vi "Initialize Message.vi"(6 "Parameters":T8[](array[typedef]) {"Base Word" format="%04d"}, 8 "error in (no error)":errorcluster, 10 "Message  Config":T1={"Time to Next Msg (4 us)"=100, "Command Config"={"Command Type"=enum."Transmit", "Terminal Address"=enum."0", "SubAddress"=enum."1", "Word Count\\Mode Code"=enum."1", "Command Data"=[]}, "Message Control"={"MC17 Time Sync"=FALSE, "Error Mask"=FALSE, "Service Request Mask"=FALSE, "Busy Mask"=FALSE, "SubSystem Flag Mask"=FALSE, "Terminal Flag Mask"=FALSE, "Reserved Mask"=FALSE, "Retry"=FALSE, "Bus A / !Bus B"=FALSE, "Self-Test Loopback"=FALSE, "Broadcast Mask"=FALSE, "EoM Interrupt"=FALSE, "Mode Code Format"=FALSE, "Broadcast Format"=FALSE, "RT-RT Format"=FALSE}}, 11 "ID":string) -> (0 "error out":errorcluster, 3 "Message out":refnum<class "Message.lvclass">)   [LabVIEW 2020, in "BCI-1553 API.lvlib" / "Message.lvclass"]
doc: "Generates a Message object that can be added to a Major Frame. Once added to a Major Frame, the Major Frame and all the Minor Frames active in it can all use this Message in their sequences.\n\nEach Message & RT-RT Message requires a unique ID within a single Major Frame."
uses:
  Message.lvclass
  TypeDefs/Simplified Parameter Data Table.ctl
  TypeDefs/Scaling Information.ctl
  TypeDefs/Message Config.ctl
  TypeDefs/Command Config.ctl
  TypeDefs/Command Type.ctl
  TypeDefs/Command Terminal Address.ctl
  TypeDefs/Command SubAddress.ctl
  TypeDefs/Command Word Count.ctl
  TypeDefs/Message Control.ctl
  TypeDefs/Parameter Table Data.ctl
  Message.lvclass/Message.ctl
  BCI-1553 API.lvlib
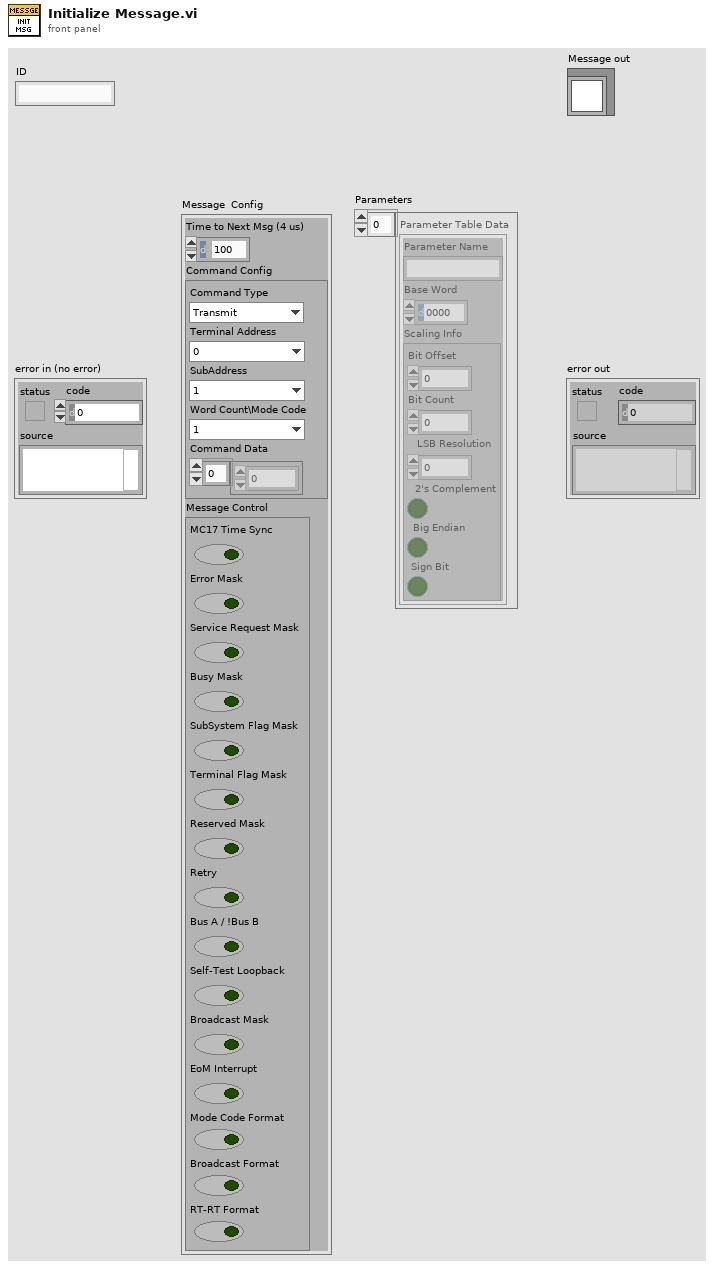
[diagram p1: front panel]
types:
  T1 = typedef "BCI-1553 API.lvlib/Message Config.ctl" = cluster{"Time to Next Msg (4 us)":u16, "Command Config":T2, "Message Control":T7}
  T2 = typedef "BCI-1553 API.lvlib/Command Config.ctl" = cluster{"Command Type":T3, "Terminal Address":T4, "SubAddress":T5, "Word Count\\Mode Code":T6, "Command Data":u16[]}
  T3 = typedef "BCI-1553 API.lvlib/Command Type.ctl" = enum16{"Transmit", "Receive"}
  T4 = typedef "BCI-1553 API.lvlib/Command Terminal Address.ctl" = enum16{"0", "1", "2", "3", "4", "5", "6", "7", "8", "9", "10", "11", "12", "13", "14", "15", "16", "17", "18", "19", "20", "21", "22", "23", "24", "25", "26", "27", "28", "29", "30", "Broadcast"}
  T5 = typedef "BCI-1553 API.lvlib/Command SubAddress.ctl" = enum16{"Mode Code", "1", "2", "3", "4", "5", "6", "7", "8", "9", "10", "11", "12", "13", "14", "15", "16", "17", "18", "19", "20", "21", "22", "23", "24", "25", "26", "27", "28", "29", "30"}
  T6 = typedef "BCI-1553 API.lvlib/Command Word Count.ctl" = enum16{"1", "2", "3", "4", "5", "6", "7", "8", "9", "10", "11", "12", "13", "14", "15", "16", "17", "18", "19", "20", "21", "22", "23", "24", "25", "26", "27", "28", "29", "30", "31", "32"}
  T7 = typedef "BCI-1553 API.lvlib/Message Control.ctl" = cluster{"MC17 Time Sync":bool, "Error Mask":bool, "Service Request Mask":bool, "Busy Mask":bool, "SubSystem Flag Mask":bool, "Terminal Flag Mask":bool, "Reserved Mask":bool, "Retry":bool, "Bus A / !Bus B":bool, "Self-Test Loopback":bool, "Broadcast Mask":bool, "EoM Interrupt":bool, "Mode Code Format":bool, "Broadcast Format":bool, "RT-RT Format":bool}
  T8 = typedef "BCI-1553 API.lvlib/Simplified Parameter Data Table.ctl" = cluster{"Parameter Name":string, "Base Word":u16, "Scaling Info":T9}
  T9 = typedef "BCI-1553 API.lvlib/Scaling Information.ctl" = cluster{"Bit Offset":i32, "Bit Count":i32, "LSB Resolution":dbl, "2's Complement":bool, "Big Endian":bool, "Sign Bit":bool}
  T10 = typedef "BCI-1553 API.lvlib/Parameter Table Data.ctl" = cluster{"Parameter Name":string, "Base Word":u16, "Address":u16, "Value":u64, "Mask":u16[], "Scaling Info":T9}
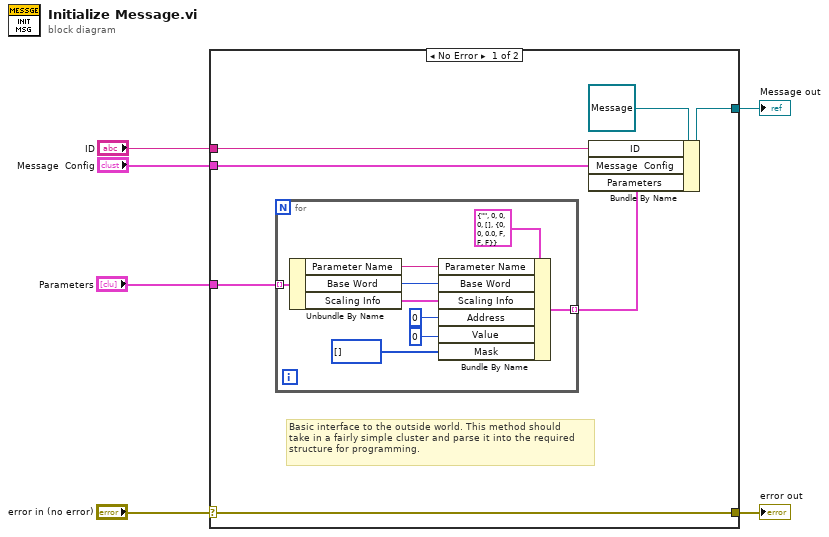
[diagram p0: block diagram]
diagram:
  n1 = case shown="No Error" "error in (no error)" {
    selector: "error in (no error)" -> [w13 w23]
    tunnel: [w13 w23] -> w5
    tunnel: [w11 _] -> w4
    tunnel: "Parameters" -> [w8 _]
    tunnel: "ID" -> [w10 _]
    tunnel: "Message  Config" -> [w9 _]
    frame No Error {
      # "Basic interface to the outside world. This method should\ntake in a fairly simple cluster and parse it into the required\nstructure for programming."
      n2 = for {
        tunnel: w8 -> [w20] mode=indexing
        tunnel: [w21] -> w7 mode=indexing
        n3 = Unbundle By Name(w20) -> ("Parameter Name"=w19:string, "Base Word"=w18:u16, "Scaling Info"=w14:T9)
        n4 = Bundle By Name(cluster=T10 {"Parameter Name"="", "Base Word"=0, "Address"=0, "Value"=0, "Mask"=[], "Scaling Info"={"Bit Offset"=0, "Bit Count"=0, "LSB Resolution"=0.0, "2's Complement"=FALSE, "Big Endian"=FALSE, "Sign Bit"=FALSE}} ("Parameter Table Data"), "Parameter Name"=w19, "Base Word"=w18, "Scaling Info"=w14, "Address"=u16 0, "Value"=u64 0, "Mask"=u16[] []) -> (w21:T10)
      }
      n5 = Bundle By Name(cluster=refnum<class "Message.lvclass"> refnum ("Message in"), "ID"=w10, "Message  Config"=w9, "Parameters"=w7) -> (w11:refnum<class "Message.lvclass">)
    }
    frame Error {
    }
  }
  "error out" <- w5
  "Message out" <- w4
